vi "Find Name.vi"(4 "abbrev":string) -> (1 "dispname":string, 2 "found?":bool)   [LabVIEW 2009, in "Magnet.lvclass"]
uses:
  Magnet.lvclass
  Global/Magnet Names.vi
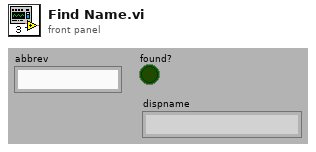
[diagram p1: front panel]
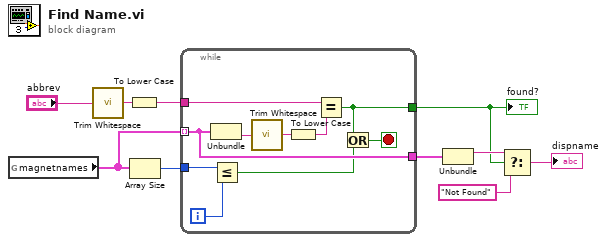
[diagram p0: block diagram]
diagram:
  n1 = global read "Magnet Names.vi" "magnetnames"() -> (w9:cluster{"dispname":string, "abbrev":string}[])
  n2 = call <vilib>:"Trim Whitespace.vi"("string"="abbrev") -> ("trimmed string"=w8:string)  [unwired: 1 in]
  n3 = To Lower Case(string=w8) -> (all lower case string=w7:string)
  n4 = Array Size(array=w9) -> (size(s)=w10:i32)
  n5 = while {
    tunnel: w10 -> [w20]
    tunnel: w9 -> [w14] mode=indexing
    tunnel: w7 -> [w15]
    tunnel: [w14] -> w5
    tunnel: [w11] -> w2
    i -> [w19]
    stop <- w12 stop-if-true
    n6 = Unbundle(w14) -> ("abbrev"=w18:string)  [unwired: 1 out]
    n7 = Less Or Equal?(x=w20, y=w19) -> (x <= y?=w13:bool)
    n8 = call <vilib>:"Trim Whitespace.vi"("string"=w18) -> ("trimmed string"=w17:string)  [unwired: 1 in]
    n9 = To Lower Case(string=w17) -> (all lower case string=w16:string)
    n10 = Equal?(x=w15, y=w16) -> (x = y?=w11:bool)
    n11 = Or(x=w11, y=w13) -> (x .or. y?=w12:bool)
  }
  "found?" <- w2
  n12 = Unbundle(w5) -> ("dispname"=w4:string)  [unwired: 1 out]
  n13 = Select(t=w4, s=w2, f="Not Found") -> (s? t:f=→"dispname":string)
